vi "test_Copy LogFile from RT cRIO.vi"(8 "error in (no error)":errorcluster, 11 "TestCase in":refnum<class "TLCD System Tests.lvclass">) -> (0 "error out":errorcluster, 3 "TestCase out":refnum<class "TLCD System Tests.lvclass">)   [LabVIEW 2019, in "TLCD System Tests.lvclass"]
uses:
  TLCD System Tests.lvclass
  <vilib>/addons/_JKI Toolkits/VI Tester/TestCase.llb/TestCase.lvclass
  TLCD Test Class/TLCD Test Class.lvclass
  b15e678b-00b4-460c-84a3-511904b6b81c.vi
  C:/Program Files (x86)/National Instruments/LabVIEW 2019/vi.lib/addons/_JKI Toolkits/VI Tester/TestCase.llb/TestCase.lvclass
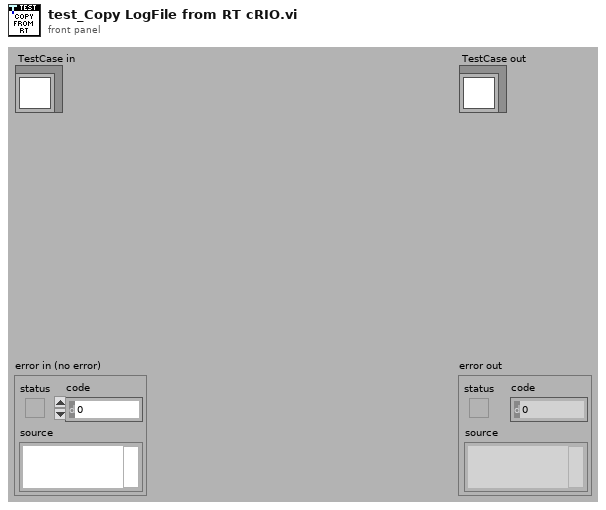
[diagram p1: front panel]
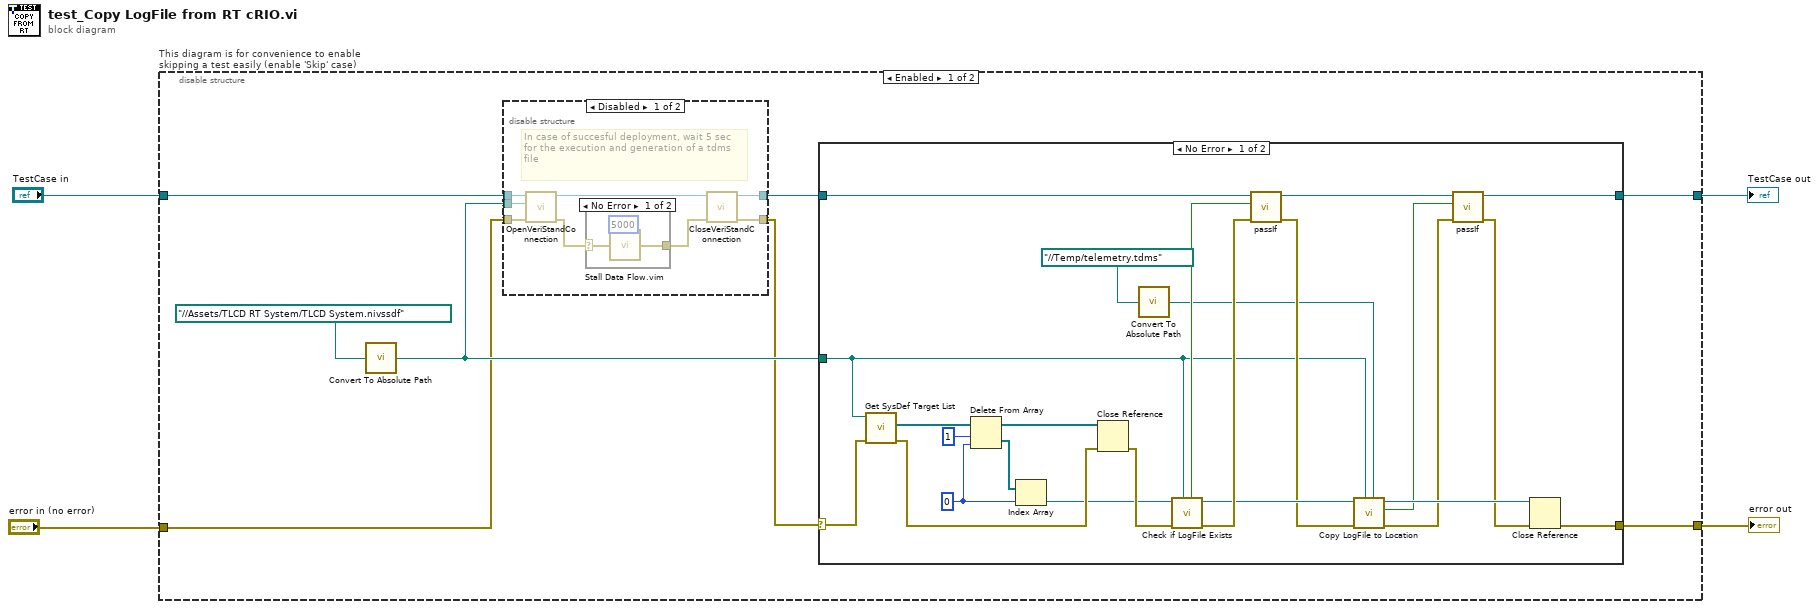
[diagram p0: block diagram]
diagram:
  n1 = disable-structure "This diagram is for convenience to enable skipping a test easily (enable 'Skip' case)" shown="Enabled" {
    disable-tunnel: "TestCase in" -> [w9 w56]
    disable-tunnel: [w10 w54] -> w1
    disable-tunnel: [w11 w55] -> w3
    disable-tunnel: "error in (no error)" -> [w7 w53]
    frame Enabled {
      n2 = call "Convert To Absolute Path.vi"("System Definition File Path"=path "../../Assets/TLCD RT System/TLCD System.nivssdf" ("relative base path")) -> ("Absolute path"=w8:path)
      n3 = disable-structure shown="Disabled" {
        disable-tunnel: w9 -> [w43 w52]
        disable-tunnel: [w42 w52] -> w6
        disable-tunnel: w8 -> [w41 _]
        disable-tunnel: w7 -> [w40 w51]
        disable-tunnel: [w39 w51] -> w5
        frame Disabled {
          # "In case of succesful deployment, wait 5 sec for the execution and generation of a tdms file"
          n4 = call-dynamic "OpenVeriStandConnection.vi"("error in (no error)"=w40, "System Definition File"=w41, "VeriStand Test Case in"=w43) -> ("error out"=w45:errorcluster, "VeriStand Test Case out"=w46:refnum<class "TLCD System Tests.lvclass">)  [unwired: 6 in, 1 out]
          n5 = case shown="No Error" w45 {
            selector: w45 -> [w49 w50]
            tunnel: [w47 w50] -> w44
            frame No Error {
              n6 = call "Stall Data Flow.vim"("value in"=w49, "milliseconds to wait"=u32 5000) -> ("value out"=w47:errorcluster)  [unwired: 1 out]
            }
            frame Error {
            }
          }
          n7 = call-dynamic "CloseVeriStandConnection.vi"("error in (no error)"=w44, "VeriStand Test Case in"=w46) -> ("error out"=w39:errorcluster, "VeriStand Test Case out"=w42:refnum<class "TLCD System Tests.lvclass">)  [unwired: 8 in]
        }
        frame Enabled {
          # "Deployment currenctly does\nnot work for Linux_x64 targets, however there is an already pregenerated file available on RT"
        }
      }
      n8 = case shown="No Error" w5 {
        selector: w5 -> [w18 w38]
        tunnel: [w36 w38] -> w11
        tunnel: [w13 w37] -> w10
        tunnel: w8 -> [w20 _]
        tunnel: w6 -> [w19 w37]
        frame No Error {
          w32 = 0 ("index")
          n9 = call "Get SysDef Target List.vi"("error in (no error)"=w18, "System Definition Path"=w20) -> ("error out"=w30:errorcluster, "Target List"=w35:refnum<k24>[])  [unwired: 8 in]
          n10 = Delete From Array(array=w35, length=1, index=w32) -> (deleted portion=w33:refnum<k24>[], array with subset deleted=w31:refnum<k24>[])
          n11 = Index Array(array=w33, index=w32) -> (element=w28:refnum<k24>)
          n12 = Close Reference(reference=w31, error in (no error)=w30) -> (error out=w29:errorcluster)
          n13 = call "Convert To Absolute Path.vi"("System Definition File Path"=path "../../Temp/telemetry.tdms" ("relative base path")) -> ("Absolute path"=w21:path)
          n14 = call "Check if LogFile Exists.vi"("System Definition Path"=w20, "error in (no error)"=w29, "Target Refnum in"=w28) -> ("error out"=w27:errorcluster, "Target Refnum out"=w25:refnum<k24>, "LogFile Exists?"=w26:bool)  [unwired: 6 in]
          n15 = call-dynamic "passIf.vi"("error in (no error)"=w27, "pass"=w26, "TestCase in"=w19) -> ("error out"=w24:errorcluster, "TestCase out"=w17:refnum<class "TLCD System Tests.lvclass">)  [unwired: 7 in]
          n16 = call "Copy LogFile to Location.vi"("Local Save path"=w21, "System Definition Path"=w20, "error in (no error)"=w24, "Target Refnum in"=w25) -> ("error out"=w15:errorcluster, "File Succesfuly copied"=w16:bool, "Target Refnum out"=w23:refnum<k24>)  [unwired: 5 in]
          n17 = call-dynamic "passIf.vi"("error in (no error)"=w15, "pass"=w16, "TestCase in"=w17) -> ("error out"=w14:errorcluster, "TestCase out"=w13:refnum<class "TLCD System Tests.lvclass">)  [unwired: 7 in]
          n18 = Close Reference(reference=w23, error in (no error)=w14) -> (error out=w36:errorcluster)
        }
        frame Error {
        }
      }
    }
    frame Disabled {
      # "skip test result while test is under development"
      n19 = call <vilib>:"skip.vi"("error in (no error)"=w53, "TestCase in"=w56) -> ("error out"=w55:errorcluster, "TestCase out"=w54:refnum<class "TLCD System Tests.lvclass">)  [unwired: 8 in]
    }
  }
  "error out" <- w3
  "TestCase out" <- w1
